vi "Setup.vi"(0 "Arduino in":refnum<class "Arduino.lvclass">, 5 "CheckPortsUpTo":i32=25, 7 "InputMarker":string, 8 "OutputMarker":string, 9 "Baud Rate":u32(ring)=9600 items=["9600"=9600, "57600"=57600], 11 "error in (no error)":errorcluster, 12 "DeviceTimeout (ms)":u32) -> (4 "Arduino out":refnum<class "Arduino.lvclass">, 15 "error out":errorcluster)   [LabVIEW 2014, in "Arduino.lvclass"]
uses:
  Arduino.lvclass
  <vilib>/Instr/_visa.llb/VISA Configure Serial Port (Instr).vi
panel:
  out "Port":string
  out "portVisa":refnum<visa-resource-name>
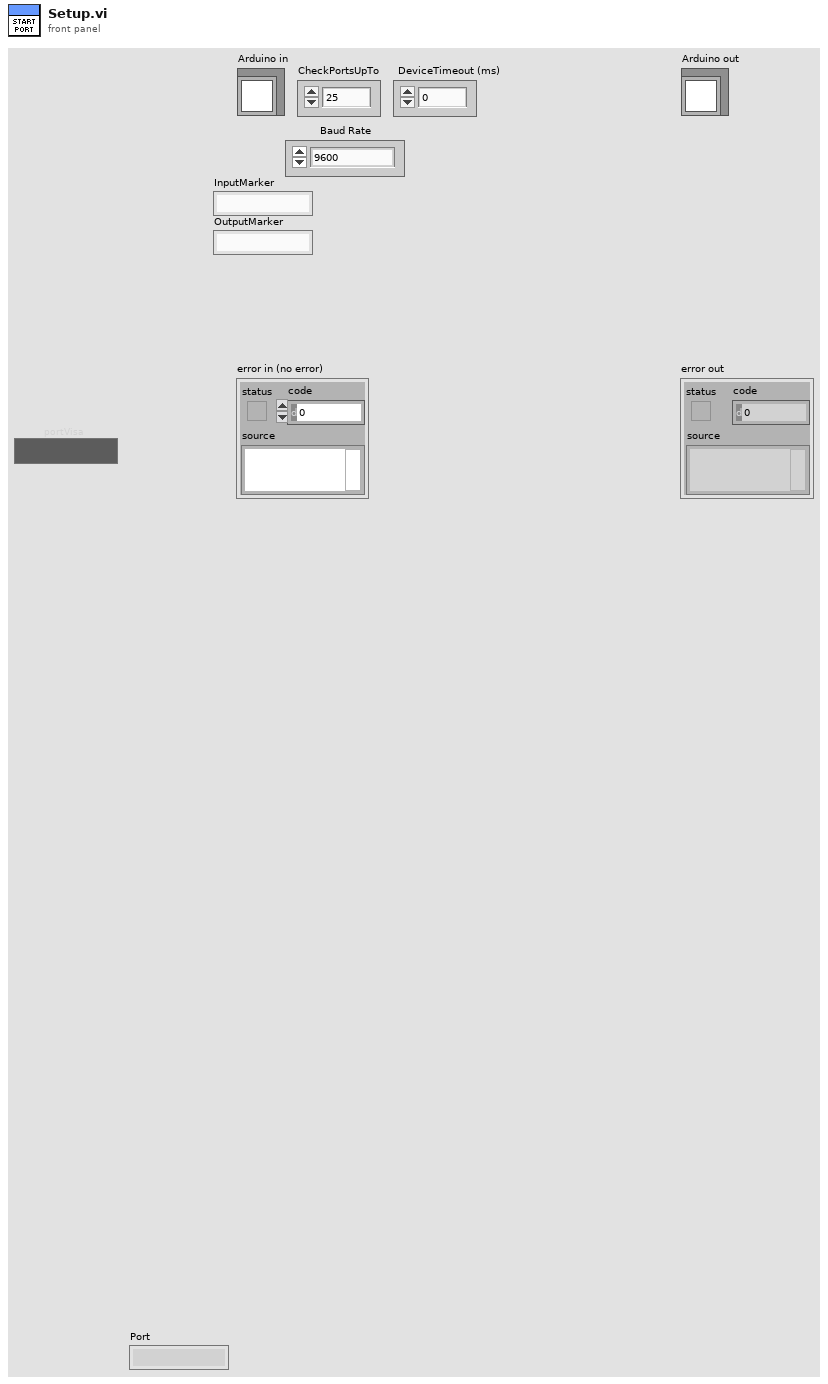
[diagram p1: front panel]
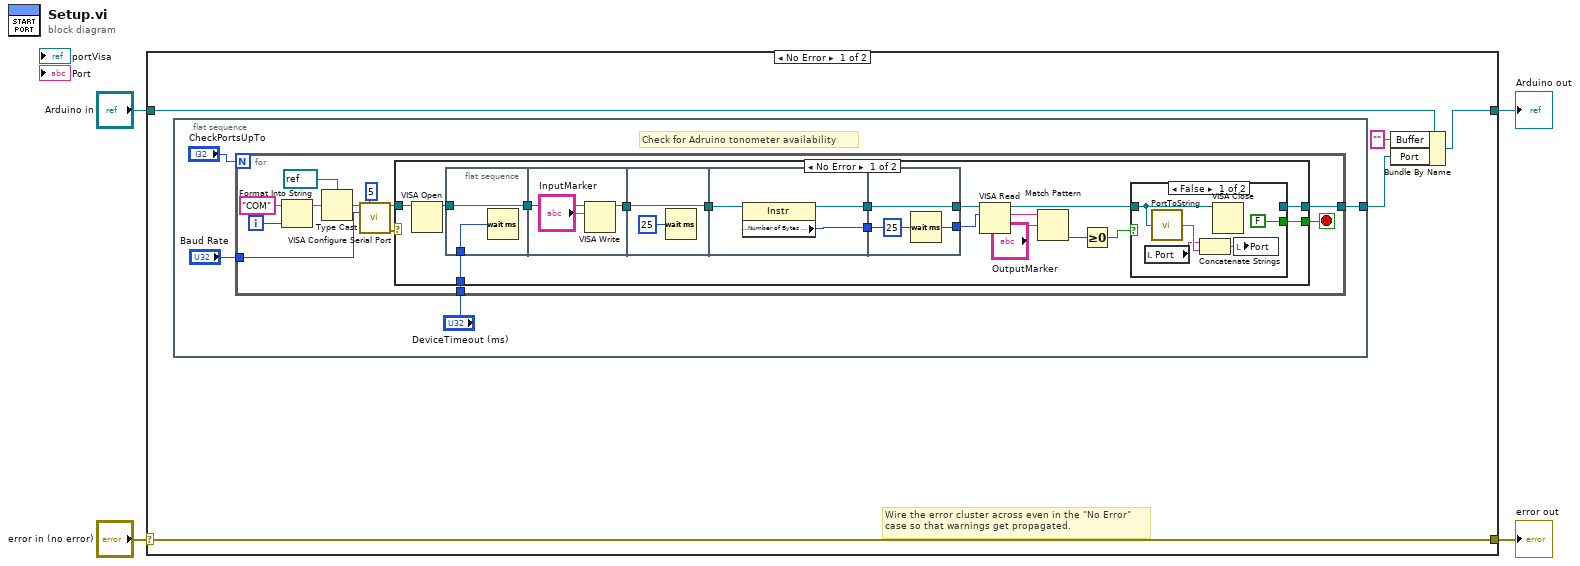
[diagram p0: block diagram]
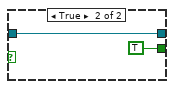
[diagram p2: hidden frame]
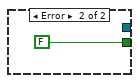
[diagram p3: hidden frame]
diagram:
  n1 = case shown="No Error" "error in (no error)" {
    selector: "error in (no error)" -> [w9 w65]
    tunnel: [w9 w65] -> w3
    tunnel: [w7 w64] -> w1
    tunnel: "Arduino in" -> [w8 w64]
    frame No Error {
      # "Wire the error cluster across even in the \"No Error\"\ncase so that warnings get propagated."
      n2 = flat-sequence {
        tunnel: [w10] -> w5
        frame #0 {
          # "Check for Adruino tonometer availability"
          n3 = for {
            N: "CheckPortsUpTo" -> [_]
            tunnel: "Baud Rate" -> [w16]
            tunnel: "DeviceTimeout (ms)" -> [w15]
            tunnel: [w14] -> w10
            i -> [w25]
            stop <- w24 stop-if-true
            n4 = Format Into String(initial string="COM", w25) -> (resulting string=w19:string)  [unwired: 2 in, 1 out]
            n5 = Type Cast(type=refnum<visa-resource-name> refnum ("portVisa"), x=w19) -> (*(type *) &x=w17:refnum<visa-resource-name>)
            n6 = call-poly "VISA Configure Serial Port"("VISA resource name"=w17, "timeout (10sec)"=u32 5, "baud rate (9600)"=w16) -> ("VISA resource name out"=w21:refnum<visa-resource-name>, "error out"=w20:errorcluster)  [unwired: 11 in]
            n7 = case shown="No Error" w20 {
              tunnel: w21 -> [w38 _]
              tunnel: [w40 FALSE] -> w24
              tunnel: w15 -> [w27 _]
              tunnel: [w26 _] -> w14
              frame No Error {
                n8 = VISA Open(VISA resource name=w38) -> (VISA resource name=w37:refnum<visa-resource-name>)  [unwired: 4 in, 1 out]
                n9 = flat-sequence {
                  tunnel: w37 -> [w51]
                  tunnel: [w51] -> w36
                  tunnel: w27 -> [w50]
                  tunnel: [w54] -> w39
                  tunnel: w36 -> [w53]
                  tunnel: [w56] -> w42
                  tunnel: w39 -> [w56]
                  tunnel: w42 -> [w59]
                  tunnel: [w58] -> w35
                  tunnel: [w57] -> w34
                  tunnel: w35 -> [w61]
                  tunnel: w34 -> [w60]
                  tunnel: [w61] -> w33
                  tunnel: [w60] -> w32
                  frame #0 {
                    n10 = Wait (ms)(milliseconds to wait=w50) -> ()  [unwired: 1 out]
                  }
                  frame #1 {
                    n11 = VISA Write(VISA resource name=w53, write buffer="InputMarker") -> (VISA resource name out=w54:refnum<visa-resource-name>)  [unwired: 1 in, 2 out]
                  }
                  frame #2 {
                    n12 = Wait (ms)(milliseconds to wait=u32 25) -> ()  [unwired: 1 out]
                  }
                  frame #3 {
                    n13 = property class="Instr"(reference=w59) -> (reference out=w58:refnum<visa-resource-name>, "Serial Settings:Number of Bytes at Serial Port"=w57:u32)  [unwired: 1 in, 1 out]
                  }
                  frame #4 {
                    n14 = Wait (ms)(milliseconds to wait=u32 25) -> ()  [unwired: 1 out]
                  }
                }
                n15 = VISA Read(VISA resource name=w33, byte count=w32) -> (VISA resource name out=w41:refnum<visa-resource-name>, read buffer=w31:string)  [unwired: 1 in, 2 out]
                n16 = Match Pattern(string=w31, regular expression="OutputMarker") -> (offset past match=w30:i32)  [unwired: 1 in, 3 out]
                n17 = Greater Or Equal To 0?(x=w30) -> (x >= 0?=w29:bool)
                n18 = case shown="False" w29 {
                  tunnel: w41 -> [w46 w48]
                  tunnel: [FALSE TRUE] -> w40
                  tunnel: [_ w48] -> w26
                  frame False {
                    n19 = local read "Port"() -> (w44:string)
                    n20 = call "PortToString.vi"("portVisa"=w46) -> ("Port"=w45:string)
                    n21 = Concatenate Strings(w44, w45) -> (w43:string)
                    n22 = VISA Close(VISA resource name=w46) -> ()  [unwired: 1 in, 1 out]
                    n23 = local write "Port"(w43) -> ()
                  }
                  frame True {
                  }
                }
              }
              frame Error {
              }
            }
          }
        }
      }
      n24 = Bundle By Name(cluster=w8, "Buffer"="", "Port"=w5) -> (w7:refnum<class "Arduino.lvclass">)
    }
    frame Error {
    }
  }
  "error out" <- w3
  "Arduino out" <- w1
